vi "NI OCR-Overlay Characters.vi"(8 "error in":errorcluster, 11 "Buffer Data In":T1={"VI Refnum"=refnum, "Src Image"=refnum, "Dst Image"=refnum, "Ctl Refnum []"=[], "Ctl Label"=[], "User Event"=refnum, "Event Registration Refnum"=refnum, "Timeout"=0, "IMAQ OCR Session"=refnum, "Objects"=[], "ROI Descriptor"={"Global Rectangle"=[], "Contours"=[]}, "Settings"={"Objects"=0, "Threshold"=128, "Reject Border"=FALSE, "Fill Holes"=FALSE, "Min Object Size"=FALSE, "Min Size"=3, "Max Object Size"=FALSE, "Max Size"=100, "Show Search Area"=FALSE, "Show Center"=TRUE, "Show Bounding Box"=TRUE}} {"Settings"."Objects" items=["Bright Objects", "Dark Objects"]; "Settings"."Threshold" min=1 max=999999999 step=1; "Settings"."Max Size" min=1 max=999999999 step=1; "Settings"."Min Size" min=1 max=999999999 step=1; "ROI Descriptor"."Contours"."Type" items=["No Selection", "Point", "Line", "Rectangle", "Oval", "Polygon", "Freehand Region", "Annulus", "Unused2", "Unused3", "Broken Line", "Freehand Line", "Rotated Rectangle"]; "Objects"."Aspect Ratio" format="%.2f"; "Objects"."Orientation" format="%.2f"; "Objects"."Area" format="%.2f"; "Objects"."Object Center"."Y" format="%.2f"; "Objects"."Object Center"."X" format="%.2f"}) -> (0 "error out":errorcluster, 3 "Buffer Data Out":T1={"VI Refnum"=refnum, "Src Image"=refnum, "Dst Image"=refnum, "Ctl Refnum []"=[], "Ctl Label"=[], "User Event"=refnum, "Event Registration Refnum"=refnum, "Timeout"=0, "IMAQ OCR Session"=refnum, "Objects"=[], "ROI Descriptor"={"Global Rectangle"=[], "Contours"=[]}, "Settings"={"Objects"=0, "Threshold"=128, "Reject Border"=FALSE, "Fill Holes"=FALSE, "Min Object Size"=FALSE, "Min Size"=3, "Max Object Size"=FALSE, "Max Size"=100, "Show Search Area"=FALSE, "Show Center"=TRUE, "Show Bounding Box"=TRUE}} {"Settings"."Objects" items=["Bright Objects", "Dark Objects"]; "Settings"."Threshold" min=1 max=999999999 step=1; "Settings"."Max Size" min=1 max=999999999 step=1; "Settings"."Min Size" min=1 max=999999999 step=1; "ROI Descriptor"."Contours"."Type" items=["No Selection", "Point", "Line", "Rectangle", "Oval", "Polygon", "Freehand Region", "Annulus", "Unused2", "Unused3", "Broken Line", "Freehand Line", "Rotated Rectangle"]; "Objects"."Aspect Ratio" format="%.2f"; "Objects"."Orientation" format="%.2f"; "Objects"."Area" format="%.2f"; "Objects"."Object Center"."Y" format="%.2f"; "Objects"."Object Center"."X" format="%.2f"})   [LabVIEW 2016]
uses:
  Data Def/NI OCR-Buffer Data.ctl
  <vilib>/vision/Image Controls.llb/IMAQ Image.ctl
  Data Def/NI OCR-User Event Data.ctl
  <vilib>/vision/OCR.llb/IMAQ OCR Session.ctl
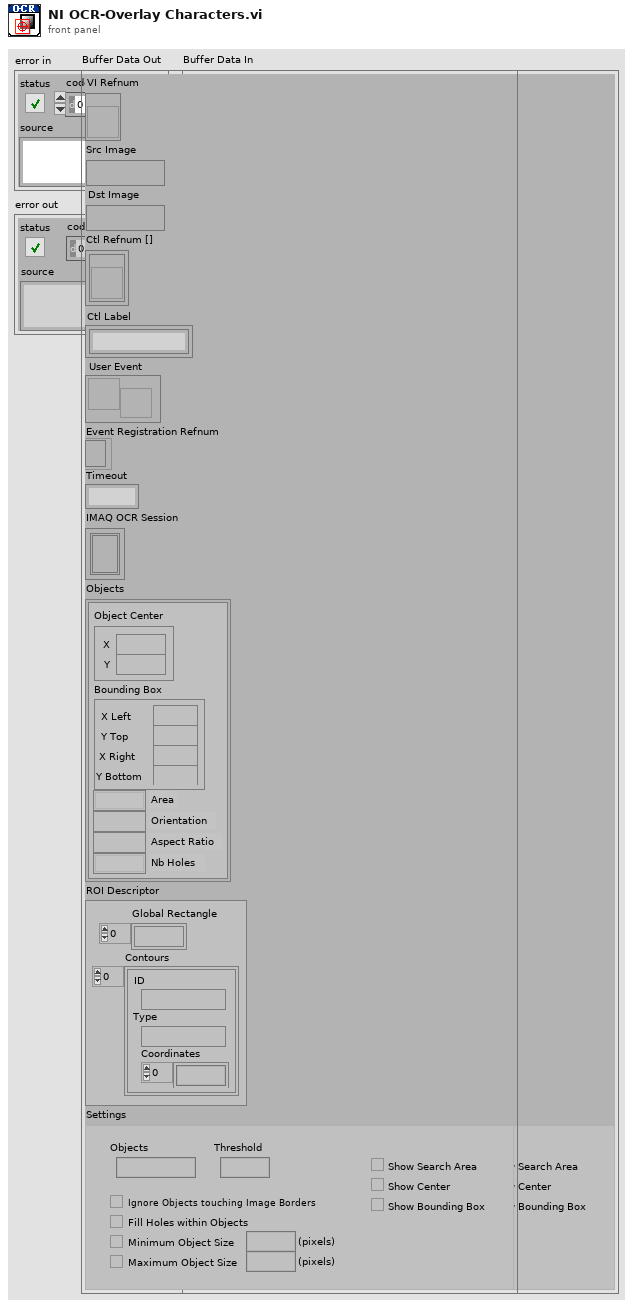
[diagram p1: front panel]
types:
  T1 = typedef "NI OCR-Buffer Data.ctl" = cluster{"VI Refnum":refnum<vi>, "Src Image":T2, "Dst Image":T2, "Ctl Refnum []":refnum<vi>[], "Ctl Label":string[], "User Event":refnum<user-event>, "Event Registration Refnum":refnum<event-registration>, "Timeout":i32, "IMAQ OCR Session":T3, "Objects":cluster{"Object Center":cluster{"X":sgl, "Y":sgl}, "Bounding Box":cluster{"X Left":i32, "Y Top":i32, "X Right":i32, "Y Bottom":i32}, "Area":sgl, "Orientation":sgl, "Aspect Ratio":sgl, "Nb Holes":i32}[], "ROI Descriptor":T4, "Settings":cluster{"Objects":u16, "Threshold":i32, "Reject Border":bool, "Fill Holes":bool, "Min Object Size":bool, "Min Size":i32, "Max Object Size":bool, "Max Size":i32, "Show Search Area":bool, "Show Center":bool, "Show Bounding Box":bool}}
  T2 = typedef "IMAQ Image.ctl" = refnum<image>
  T3 = typedef "IMAQ OCR Session.ctl" = refnum<k1>
  T4 = typedef "ROI Descriptor" = cluster{"Global Rectangle":i32[], "Contours":cluster{"ID":enum32{"External", "Internal"}, "Type":u32, "Coordinates":i32[]}[]}
  T5 = cluster{"Object Center":cluster{"X":sgl, "Y":sgl}, "Bounding Box":cluster{"X Left":i32, "Y Top":i32, "X Right":i32, "Y Bottom":i32}, "Area":sgl, "Orientation":sgl, "Aspect Ratio":sgl, "Nb Holes":i32}[]
  T6 = cluster{"[0]":sgl, "[1]":sgl, "[2]":sgl, "[3]":sgl}
  T7 = cluster{"X Left":i32, "Y Top":i32, "X Right":i32, "Y Bottom":i32}
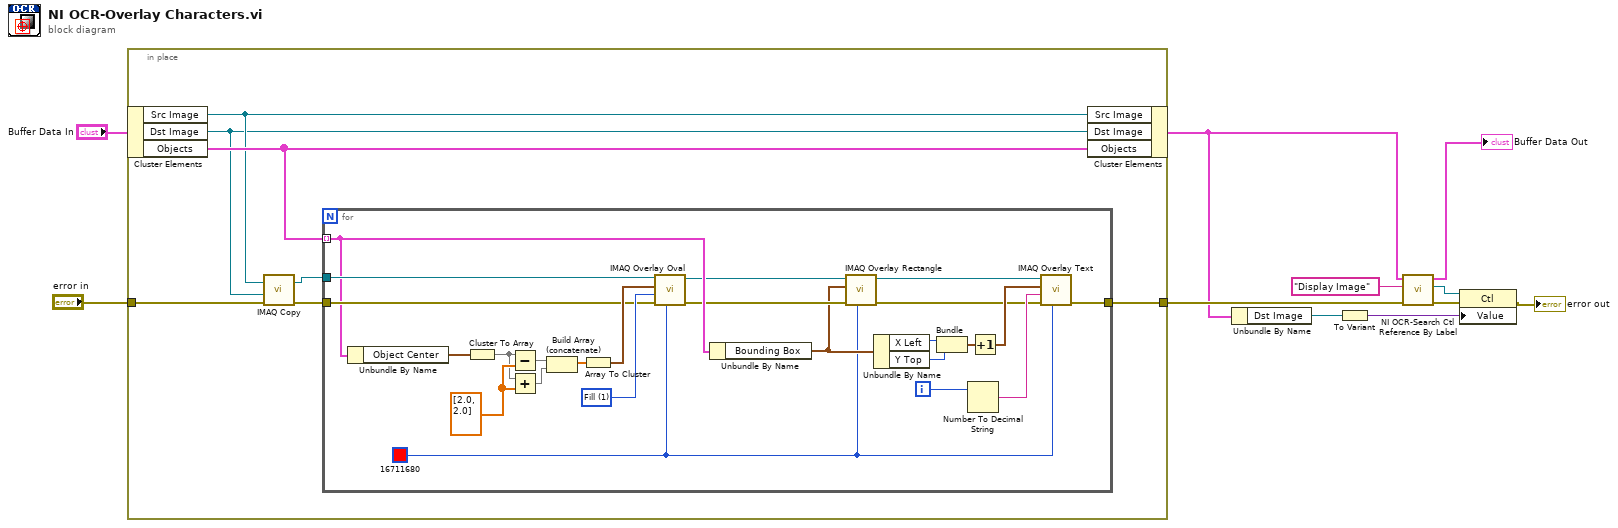
[diagram p0: block diagram]
diagram:
  n1 = in-place {
    in-place-border: "error in" -> [w16]
    in-place-border: [w17] -> w5
    n2 = in-place-cluster #1("Buffer Data In") -> ("Src Image"=w15:T2, "Dst Image"=w14:T2, "Objects"=w18:T5)
    n3 = call "IMAQ Copy"("error in (no error)"=w16, "Image Dst"=w14, "Image Src"=w15) -> ("error out"=w13:errorcluster, "Image Dst Out"=w12:T2)  [unwired: 3 in]
    n4 = for {
      tunnel: w12 -> [w37]
      tunnel: w18 -> [w34] mode=indexing
      tunnel: w13 -> [w35]
      tunnel: [w21] -> w17
      i -> [w24]
      w22 = u32 16711680 ("Color")
      w38 = u32 1 items=["Frame", "Fill"] ("Drawing Mode (Frame)")
      w39 = sgl[] [2.0, 2.0] ("y")
      n5 = Unbundle By Name(w34) -> ("Object Center"=w36:cluster{"X":sgl, "Y":sgl})
      n6 = Cluster To Array(cluster=w36) -> (array=w20:sgl[])
      n7 = Subtract(x=w20, y=w39) -> (x-y=w42:sgl[])
      n8 = Add(x=w20, y=w39) -> (x+y=w19:sgl[])
      n9 = Build Array (concatenate)(w42, w19) -> (w41:sgl[])
      n10 = Array To Cluster(array=w41) -> (cluster=w40:T6)
      n11 = call "IMAQ Overlay Oval"("Color"=w22, "error in (no error)"=w35, "Drawing Mode (Frame)"=w38, "Bounding Rectangle"=w40, "Image"=w37) -> ("error out"=w28:errorcluster, "Image Out"=w27:T2)  [unwired: 1 in, 4 out]
      n12 = Unbundle By Name(w34) -> ("Bounding Box"=w26:T7)
      n13 = call "IMAQ Overlay Rectangle"("Color"=w22, "error in (no error)"=w28, "Rectangle"=w26, "Image"=w27) -> ("error out"=w23:errorcluster, "Image Out"=w32:T2)  [unwired: 2 in, 4 out]
      n14 = Unbundle By Name(w26) -> ("X Left"=w31:i32, "Y Top"=w30:i32)
      n15 = Bundle("X Left"=w31, "Y Top"=w30) -> (w25:cluster{"X Left":i32, "Y Top":i32})  [unwired: 1 out]
      n16 = Number To Decimal String(number=w24) -> (decimal integer string=w33:string)  [unwired: 1 out]
      n17 = Increment(x=w25) -> (x+1=w29:cluster{"X Left":i32, "Y Top":i32})
      n18 = call "IMAQ Overlay Text"("Text Color (black)"=w22, "error in (no error)"=w23, "String"=w33, "Origin"=w29, "Image"=w32) -> ("error out"=w21:errorcluster)  [unwired: 3 in, 3 out]
    }
    n19 = in-place-cluster #1("Src Image"=w15, "Dst Image"=w14, "Objects"=w18) -> (w2:T1)
  }
  n20 = Unbundle By Name(w2) -> ("Dst Image"=w1:T2)
  n21 = To Variant(anything=w1) -> (Variant=w6:variant)
  n22 = call "NI OCR-Search Ctl Reference By Label.vi"("error in"=w5, "Ctl Label"="Display Image", "Buffer Data In"=w2) -> ("error out"=w8:errorcluster, "Ctl Refnum"=w7:refnum<vi>, "Buffer Data Out"=→"Buffer Data Out":T1)  [unwired: 5 in, 1 out]
  n23 = property class="Ctl"(reference=w7, error in=w8, "Value"=w6) -> (error out=→"error out":errorcluster)  [unwired: 1 out]
